vi "close.vi"(8 "error in (no error)":errorcluster, 11 "Lakeshore 336 in":refnum<class "Lakeshore 336.lvclass">) -> (0 "error out":errorcluster, 3 "Lakeshore 336 out":refnum<class "Lakeshore 336.lvclass">)   [LabVIEW 2022 SP3, in "Lakeshore 336.lvclass"]
uses:
  Lakeshore 336.lvclass
  Lakeshore 336.lvclass/Lakeshore 336.ctl
  Temp Control.lvclass
  <instrlib>/Lake Shore 336/Lake Shore 336.lvlib
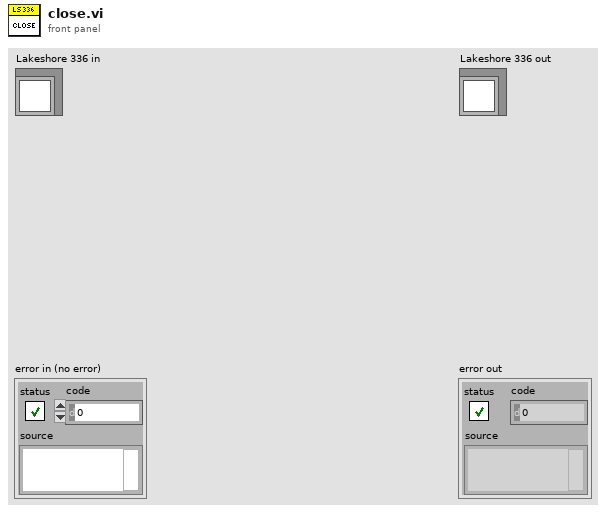
[diagram p1: front panel]
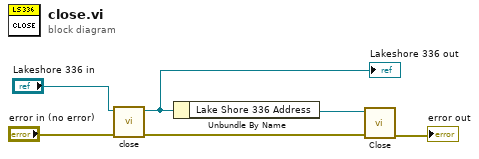
[diagram p0: block diagram]
diagram:
  n1 = call-parent <instrlib>:"close.vi"("error in (no error)"="error in (no error)", "Temp Control in"="Lakeshore 336 in") -> ("error out"=w3:errorcluster, "Temp Control out"=w1:refnum<class "Lakeshore 336.lvclass">)  [unwired: 8 in]
  "Lakeshore 336 out" <- w1
  n2 = Unbundle By Name(w1) -> ("Lake Shore 336 Address"=w4:refnum<visa-resource-name>)
  n3 = call <instrlib>:"Close.vi"("error in (no error)"=w3, "VISA resource name"=w4) -> ("error out"=→"error out":errorcluster)  [unwired: 9 in]
